vi "Obtain NI Settings UL.vi"(11 "Cluster INFO":T1={"Coefficenti P2"={"Af"=0.0, "Bf"=0.0, "Cf"=0.0, "Df"=0.0, "Ef"=0.0, "Ff"=0.0, "Gf"=0.0, "Hf"=0.0, "Jf"=0.0, "Kf"=0.0, "If"=0.0, "Ar"=0.0, "Br"=0.0, "Cr"=0.0, "Dr"=0.0, "Er"=0.0, "Fr"=0.0, "Gr"=0.0, "Hr"=0.0, "Jr"=0.0, "Kr"=0.0, "Ir"=0.0}, "Cluster settaggi wattmetro"={"Wattmetro"=enum."No Selection", "Alimentazione"=enum."Radio Selection 1"}, "SET RPM"=0.0, "SET TEMP"=0.0, "IMPOSTAZIONI INGRESSI UL"={"SALVA"=FALSE, "CARICA"=FALSE, "APPLICA"=FALSE, "Q1"={"Range"=0.0, "Offset"=0.0, "Medie"=0}, "Q2"={"Range"=0.0, "Offset"=0.0, "Medie"=0}, "Q3"={"Range"=0.0, "Offset"=0.0, "Medie"=0}, "P1"={"Range"=0.0, "Offset"=0.0, "Medie"=0}, "P2"={"Range"=0.0, "Offset"=0.0, "Medie"=0}, "P3"={"Range"=0.0, "Offset"=0.0, "Medie"=0}, "N"={"Range"=0.0, "Offset"=0.0, "Medie"=0}, "Tq"={"Range"=0.0, "Offset"=0.0, "Medie"=0}, "T"={"Range"=0.0, "Offset"=0.0, "Medie"=0}, "PORTATA PRINCIPALE"=0, "PORTATA SECONDARIA"=0, "PRESSIONE ASPIRAZIONE"=0, "PRESSIONE MANDATA"=0, "RPM"=0, "differenziale?"=FALSE}, "IMPOSTAZIONI INGRESSI NM"={"SALVA"=FALSE, "CARICA"=FALSE, "APPLICA"=FALSE, "Q1"={"Range"=0.0, "Offset"=0.0, "Medie"=0}, "Q2"={"Range"=0.0, "Offset"=0.0, "Medie"=0}, "Q3"={"Range"=0.0, "Offset"=0.0, "Medie"=0}, "Q4"={"Range"=0.0, "Offset"=0.0, "Medie"=0}, "Q5"={"Range"=0.0, "Offset"=0.0, "Medie"=0}, "Q6"={"Range"=0.0, "Offset"=0.0, "Medie"=0}, "Q7"={"Range"=0.0, "Offset"=0.0, "Medie"=0}, "Q8"={"Range"=0.0, "Offset"=0.0, "Medie"=0}, "Q9"={"Range"=0.0, "Offset"=0.0, "Medie"=0}, "Q10"={"Range"=0.0, "Offset"=0.0, "Medie"=0}, "P1"={"Range"=0.0, "Offset"=0.0, "Medie"=0}, "P2"={"Range"=0.0, "Offset"=0.0, "Medie"=0}, "P3"={"Range"=0.0, "Offset"=0.0, "Medie"=0}, "P4"={"Range"=0.0, "Offset"=0.0, "Medie"=0}, "P5"={"Range"=0.0, "Offset"=0.0, "Medie"=0}, "P6"={"Range"=0.0, "Offset"=0.0, "Medie"=0}, "P7"={"Range"=0.0, "Offset"=0.0, "Medie"=0}, "P8"={"Range"=0.0, "Offset"=0.0, "Medie"=0}, "P9"={"Range"=0.0, "Offset"=0.0, "Medie"=0}, "P10"={"Range"=0.0, "Offset"=0.0, "Medie"=0}, "N1(T)"={"Range"=0.0, "Offset"=0.0, "Medie"=0}, "N2(T)"={"Range"=0.0, "Offset"=0.0, "Medie"=0}, "N3(T)"={"Range"=0.0, "Offset"=0.0, "Medie"=0}, "Tq1"={"Range"=0.0, "Offset"=0.0, "Medie"=0}, "Tq2"={"Range"=0.0, "Offset"=0.0, "Medie"=0}, "Tq3"={"Range"=0.0, "Offset"=0.0, "Medie"=0}, "RM1"={"Range"=0.0, "Offset"=0.0, "Medie"=0}, "RM2"={"Range"=0.0, "Offset"=0.0, "Medie"=0}, "RM3"={"Range"=0.0, "Offset"=0.0, "Medie"=0}, "T1"={"Range"=0.0, "Offset"=0.0, "Medie"=0}, "T2"={"Range"=0.0, "Offset"=0.0, "Medie"=0}, "T3"={"Range"=0.0, "Offset"=0.0, "Medie"=0}, "T4"={"Range"=0.0, "Offset"=0.0, "Medie"=0}, "T5"={"Range"=0.0, "Offset"=0.0, "Medie"=0}, "T6"={"Range"=0.0, "Offset"=0.0, "Medie"=0}, "T7"={"Range"=0.0, "Offset"=0.0, "Medie"=0}, "T8"={"Range"=0.0, "Offset"=0.0, "Medie"=0}, "Liv."={"Range"=0.0, "Offset"=0.0, "Medie"=0}, "Pbar"={"Range"=0.0, "Offset"=0.0, "Medie"=0}, "PORTATA\nPRINCIPALE"=0, "PORTATA\nSECONDARIA"=0, "PRESSIONE\nASPIRAZIONE"=0, "PRESSIONE\nMANDATA"=0, "RPM"=0, "differenziale?"=FALSE}, "Costanti collaudo"={"P [bar]"=0.0, "T amb. [°C]"=0.0, "Umidità [%]"=0.0}, "Condizione P2"=enum."Radio Selection 1", "Array linee"=[{"portata"=0, "Hasp"=0, "Hmand"=1, "Torsiometro"=0, "rpm"=0, "Hdiff?"=FALSE, "T amb"=0, "Indici valvole"=[0, 1], "Nome"="Elettropompa", "Sommersa?"=FALSE}, {"portata"=1, "Hasp"=0, "Hmand"=0, "Torsiometro"=0, "rpm"=0, "Hdiff?"=FALSE, "T amb"=0, "Indici valvole"=[0, 1], "Nome"="Sommersa", "Sommersa?"=TRUE}], "Array valvole linee avvio/fermata"=[], "Linea selezionata"=0.0, "Tolleranze croci"={"Q"=0.0, "Htot"=0.0, "Ptot"=0.0, "EtaP"=0.0}, "Sett T e R"={"Tamb[°C]"=0.0, "Ru-w"=0.0, "Rmarcia"=0.0, "Raux"=0.0, "Tamb Freddo[°C]"=0.0, "Ru-w freddo"=0.0, "Rmarcia freddo"=0.0, "Raux freddop"=0.0, "TC1"=0.0, "TC2"=0.0, "TC3"=0.0, "TC4"=0.0, "TC5"=0.0, "TC6"=0.0, "TC7"=0.0, "TC8"=0.0}, "Nomi valvole prop sistema"=[], "Calcolo P2"=enum."Torsiometro", "Rendimento motore"=0.0, "curva rendimento"=[], "Coeff motore"={"a5"=0.0, "a4"=0.0, "a3"=0.0, "a2"=0.0, "a1"=0.0, "a0"=0.0, "P1max"=0.0, "P1min"=0.0}} {"IMPOSTAZIONI INGRESSI NM"."T8"."Medie" min=1 step=1; "IMPOSTAZIONI INGRESSI NM"."T7"."Medie" min=1 step=1; "IMPOSTAZIONI INGRESSI NM"."T6"."Medie" min=1 step=1; "IMPOSTAZIONI INGRESSI NM"."T5"."Medie" min=1 step=1; "IMPOSTAZIONI INGRESSI NM"."T4"."Medie" min=1 step=1; "IMPOSTAZIONI INGRESSI NM"."T3"."Medie" min=1 step=1; "IMPOSTAZIONI INGRESSI NM"."RM3"."Medie" min=1 step=1; "IMPOSTAZIONI INGRESSI NM"."Tq3"."Medie" min=1 step=1; "IMPOSTAZIONI INGRESSI NM"."Tq2"."Medie" min=1 step=1; "IMPOSTAZIONI INGRESSI NM"."N3(T)"."Medie" min=1 step=1; "IMPOSTAZIONI INGRESSI NM"."N2(T)"."Medie" min=1 step=1; "IMPOSTAZIONI INGRESSI NM"."P10"."Medie" min=1 step=1; "IMPOSTAZIONI INGRESSI NM"."P9"."Medie" min=1 step=1; "IMPOSTAZIONI INGRESSI NM"."P8"."Medie" min=1 step=1; "IMPOSTAZIONI INGRESSI NM"."P7"."Medie" min=1 step=1; "IMPOSTAZIONI INGRESSI NM"."P6"."Medie" min=1 step=1; "IMPOSTAZIONI INGRESSI NM"."P5"."Medie" min=1 step=1; "IMPOSTAZIONI INGRESSI NM"."Q10"."Medie" min=1 step=1; "IMPOSTAZIONI INGRESSI NM"."Q9"."Medie" min=1 step=1; "IMPOSTAZIONI INGRESSI NM"."Q8"."Medie" min=1 step=1; "IMPOSTAZIONI INGRESSI NM"."Q7"."Medie" min=1 step=1; "IMPOSTAZIONI INGRESSI NM"."Q6"."Medie" min=1 step=1; "IMPOSTAZIONI INGRESSI NM"."Q5"."Medie" min=1 step=1; "IMPOSTAZIONI INGRESSI NM"."Pbar"."Medie" min=1 step=1; "IMPOSTAZIONI INGRESSI NM"."Liv."."Medie" min=1 step=1; "IMPOSTAZIONI INGRESSI NM"."RM2"."Medie" min=1 step=1; "IMPOSTAZIONI INGRESSI NM"."RM1"."Medie" min=1 step=1; "IMPOSTAZIONI INGRESSI NM"."T2"."Medie" min=1 step=1; "IMPOSTAZIONI INGRESSI NM"."P4"."Medie" min=1 step=1; "IMPOSTAZIONI INGRESSI NM"."Q4"."Medie" min=1 step=1; "IMPOSTAZIONI INGRESSI NM"."RPM" items=["TESTO", "TORSIOMETRO", "OTTICA"]; "IMPOSTAZIONI INGRESSI NM"."PRESSIONE\nMANDATA" items=["P1", "P2", "P3", "P4"]; "IMPOSTAZIONI INGRESSI NM"."PRESSIONE\nASPIRAZIONE" items=["P1", "P2", "P3", "P4"]; "IMPOSTAZIONI INGRESSI NM"."PORTATA\nSECONDARIA" items=["Q1", "Q2", "Q3", "Q4"]; "IMPOSTAZIONI INGRESSI NM"."PORTATA\nPRINCIPALE" items=["LINEA ELETTROPOMPA", "LINEA SOMMERSA"]; "IMPOSTAZIONI INGRESSI NM"."T1"."Medie" min=1 step=1; "IMPOSTAZIONI INGRESSI NM"."Tq1"."Medie" min=1 step=1; "IMPOSTAZIONI INGRESSI NM"."N1(T)"."Medie" min=1 step=1; "IMPOSTAZIONI INGRESSI NM"."P3"."Medie" min=1 step=1; "IMPOSTAZIONI INGRESSI NM"."P2"."Medie" min=1 step=1; "IMPOSTAZIONI INGRESSI NM"."P1"."Medie" min=1 step=1; "IMPOSTAZIONI INGRESSI NM"."Q3"."Medie" min=1 step=1; "IMPOSTAZIONI INGRESSI NM"."Q2"."Medie" min=1 step=1; "IMPOSTAZIONI INGRESSI NM"."Q1"."Medie" min=1 step=1; "IMPOSTAZIONI INGRESSI UL"."RPM" items=["TESTO", "TORSIOMETRO", "OTTICA"]; "IMPOSTAZIONI INGRESSI UL"."PRESSIONE MANDATA" items=["P1", "P2", "P3"]; "IMPOSTAZIONI INGRESSI UL"."PRESSIONE ASPIRAZIONE" items=["P1", "P2", "P3"]; "IMPOSTAZIONI INGRESSI UL"."PORTATA SECONDARIA" items=["Q1", "Q2", "Q3"]; "IMPOSTAZIONI INGRESSI UL"."PORTATA PRINCIPALE" items=["Q1", "Q2", "Q3"]; "IMPOSTAZIONI INGRESSI UL"."T"."Medie" min=1 step=1; "IMPOSTAZIONI INGRESSI UL"."Tq"."Medie" min=1 step=1; "IMPOSTAZIONI INGRESSI UL"."N"."Medie" min=1 step=1; "IMPOSTAZIONI INGRESSI UL"."P3"."Medie" min=1 step=1; "IMPOSTAZIONI INGRESSI UL"."P2"."Medie" min=1 step=1; "IMPOSTAZIONI INGRESSI UL"."P1"."Medie" min=1 step=1; "IMPOSTAZIONI INGRESSI UL"."Q3"."Medie" min=1 step=1; "IMPOSTAZIONI INGRESSI UL"."Q2"."Medie" min=1 step=1; "IMPOSTAZIONI INGRESSI UL"."Q1"."Medie" min=1 step=1}) -> (1 "Campioni medie":u8[](array[numeric]), 3 "Array Settings":dbl[](array[numeric]))   [LabVIEW 2016]
uses:
  TypeDef/Cluster INFO.ctl
  TypeDef/WT SELECTION.ctl
  TypeDef/ALIM SELECTION.ctl
  TypeDef/cDAQ Settings UL.ctl
  TypeDef/SETUP INGRESSO.ctl
  TypeDef/cDAQ Settings NM.ctl
  TypeDef/Definizione linea.ctl
  TypeDef/sett T e R.ctl
panel:
  # "Freddo"
  # "Regime"
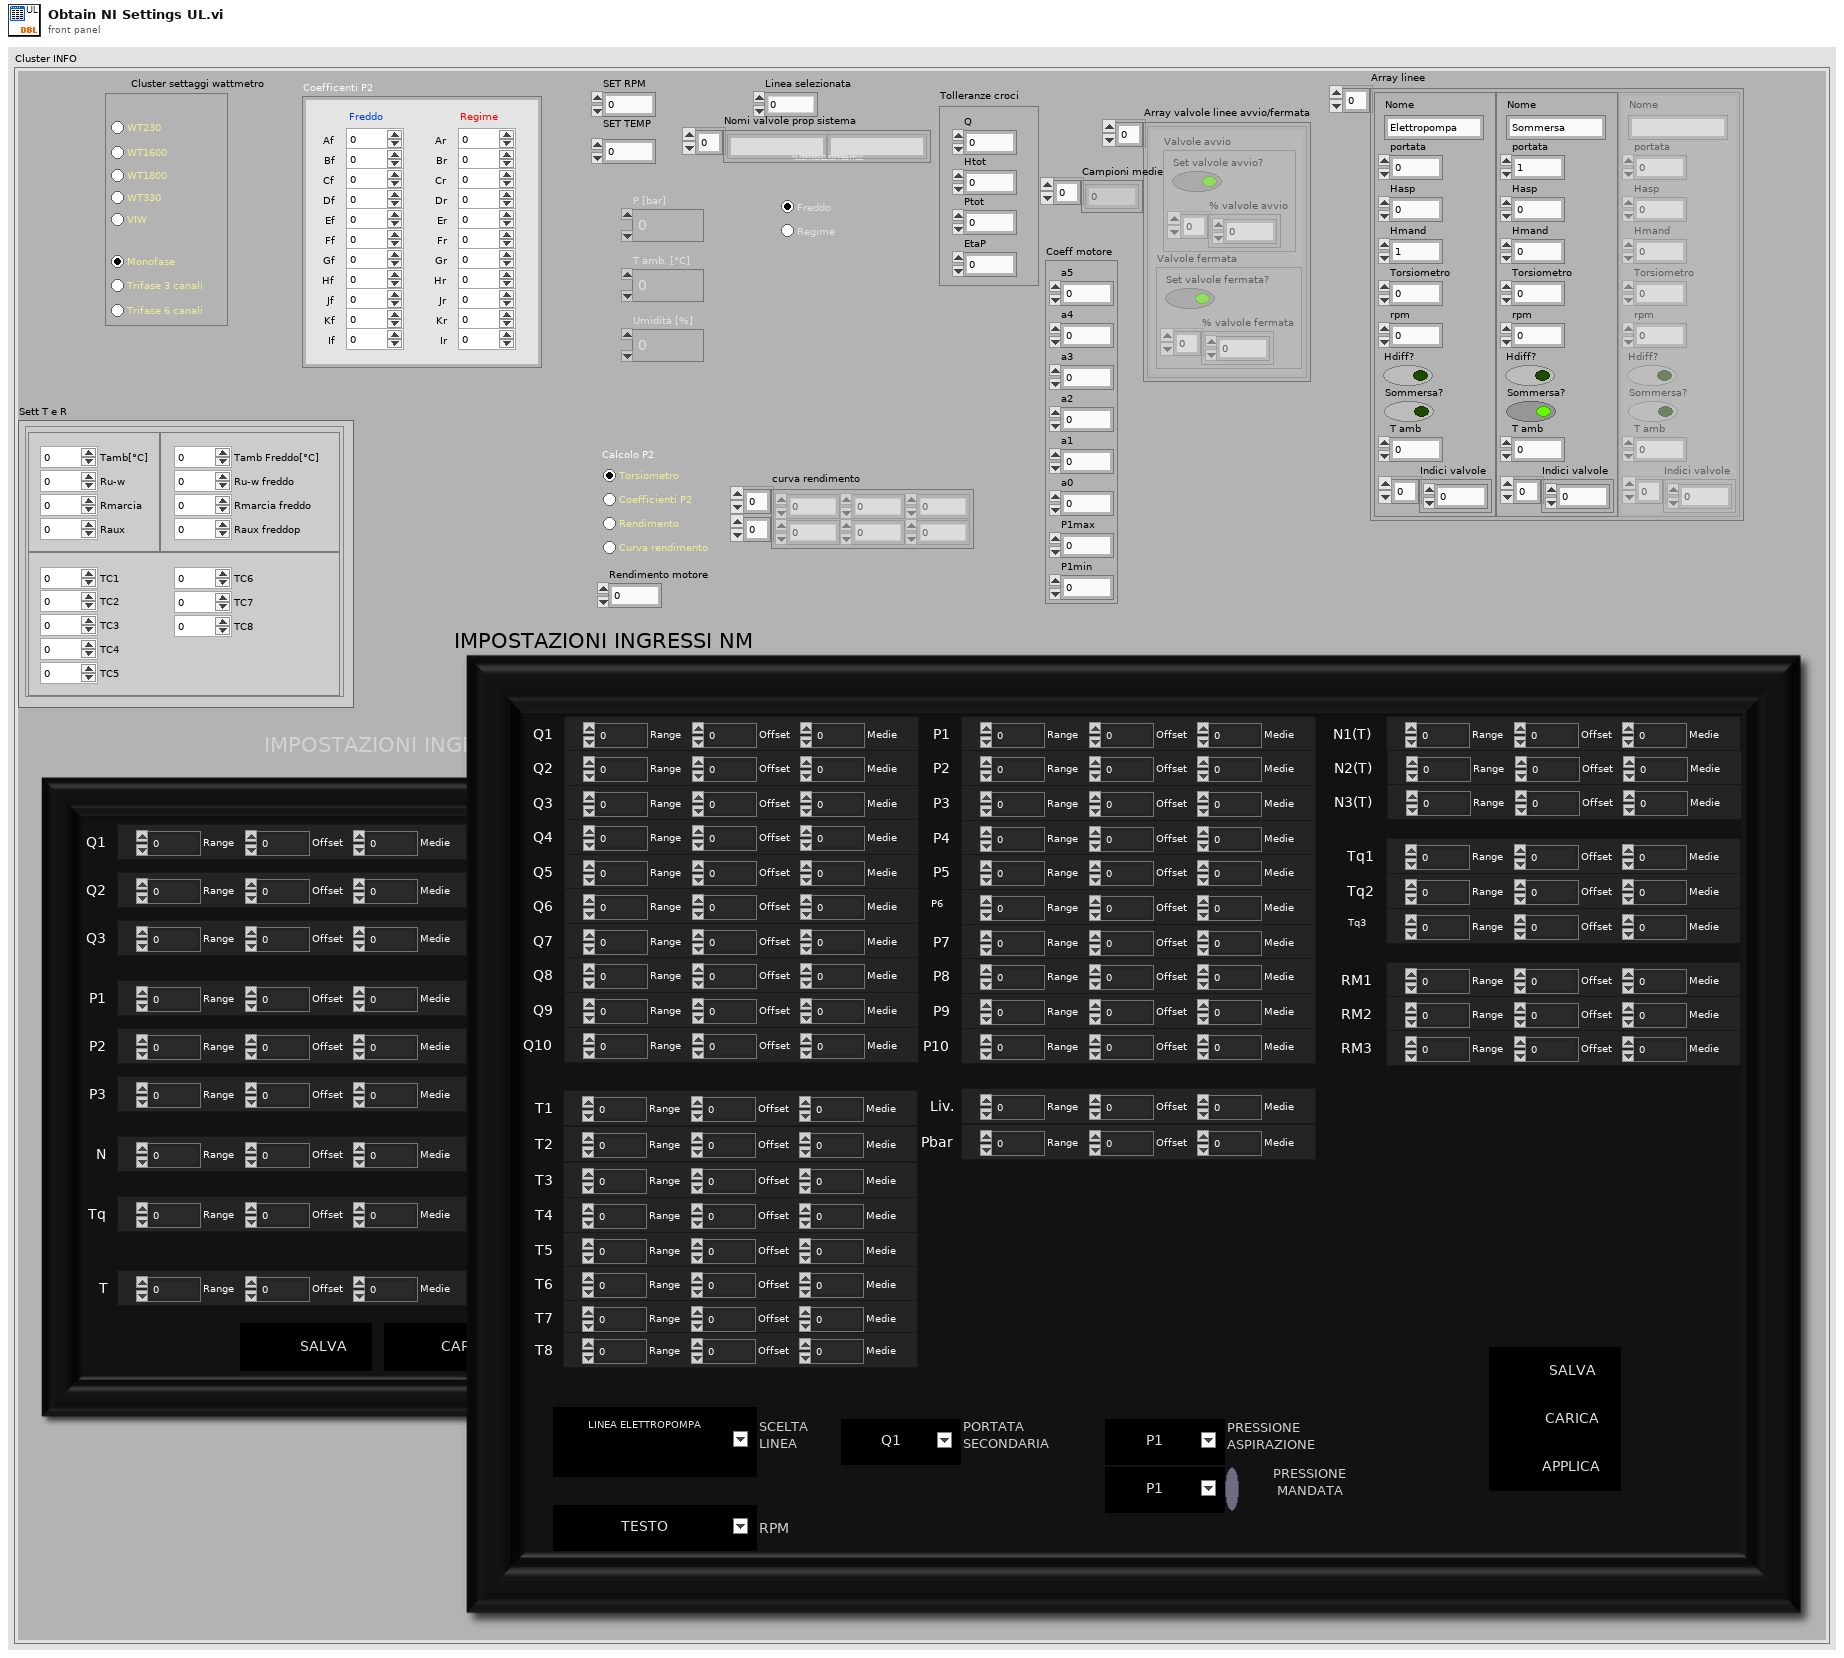
[diagram p1: front panel]
types:
  T1 = typedef "Cluster INFO.ctl" = cluster{"Coefficenti P2":cluster{"Af":dbl, "Bf":dbl, "Cf":dbl, "Df":dbl, "Ef":dbl, "Ff":dbl, "Gf":dbl, "Hf":dbl, "Jf":dbl, "Kf":dbl, "If":dbl, "Ar":dbl, "Br":dbl, "Cr":dbl, "Dr":dbl, "Er":dbl, "Fr":dbl, "Gr":dbl, "Hr":dbl, "Jr":dbl, "Kr":dbl, "Ir":dbl}, "Cluster settaggi wattmetro":cluster{"Wattmetro":T2, "Alimentazione":T3}, "SET RPM":dbl, "SET TEMP":dbl, "IMPOSTAZIONI INGRESSI UL":T4, "IMPOSTAZIONI INGRESSI NM":T6, "Costanti collaudo":cluster{"P [bar]":dbl, "T amb. [°C]":dbl, "Umidità [%]":dbl}, "Condizione P2":enum32{"Radio Selection 1", "Radio Selection 2"}, "Array linee":T7[], "Array valvole linee avvio/fermata":cluster{"Valvole avvio":cluster{"Set valvole avvio?":bool, "% valvole avvio":dbl[]}, "Valvole fermata":cluster{"Set valvole fermata?":bool, "% valvole fermata":dbl[]}}[], "Linea selezionata":dbl, "Tolleranze croci":cluster{"Q":dbl, "Htot":dbl, "Ptot":dbl, "EtaP":dbl}, "Sett T e R":T8, "Nomi valvole prop sistema":string[], "Calcolo P2":enum32{"Torsiometro", "coeff p2", "Rendimento", "Curva rend"}, "Rendimento motore":dbl, "curva rendimento":dbl[][], "Coeff motore":cluster{"a5":dbl, "a4":dbl, "a3":dbl, "a2":dbl, "a1":dbl, "a0":dbl, "P1max":dbl, "P1min":dbl}}
  T2 = typedef "WT SELECTION.ctl" = enum32{"No Selection", "WT230", "WT1600", "WT1800", "WT330", "VIW"}
  T3 = typedef "ALIM SELECTION.ctl" = enum32{"Radio Selection 1", "Radio Selection 2", "Radio Selection 3"}
  T4 = typedef "cDAQ Settings UL.ctl" = cluster{"SALVA":bool, "CARICA":bool, "APPLICA":bool, "Q1":T5, "Q2":T5, "Q3":T5, "P1":T5, "P2":T5, "P3":T5, "N":T5, "Tq":T5, "T":T5, "PORTATA PRINCIPALE":u16, "PORTATA SECONDARIA":u16, "PRESSIONE ASPIRAZIONE":u16, "PRESSIONE MANDATA":u16, "RPM":u16, "differenziale?":bool}
  T5 = typedef "SETUP INGRESSO.ctl" = cluster{"Range":dbl, "Offset":dbl, "Medie":u8}
  T6 = typedef "cDAQ Settings NM.ctl" = cluster{"SALVA":bool, "CARICA":bool, "APPLICA":bool, "Q1":T5, "Q2":T5, "Q3":T5, "Q4":T5, "Q5":T5, "Q6":T5, "Q7":T5, "Q8":T5, "Q9":T5, "Q10":T5, "P1":T5, "P2":T5, "P3":T5, "P4":T5, "P5":T5, "P6":T5, "P7":T5, "P8":T5, "P9":T5, "P10":T5, "N1(T)":T5, "N2(T)":T5, "N3(T)":T5, "Tq1":T5, "Tq2":T5, "Tq3":T5, "RM1":T5, "RM2":T5, "RM3":T5, "T1":T5, "T2":T5, "T3":T5, "T4":T5, "T5":T5, "T6":T5, "T7":T5, "T8":T5, "Liv.":T5, "Pbar":T5, "PORTATA\nPRINCIPALE":u16, "PORTATA\nSECONDARIA":u16, "PRESSIONE\nASPIRAZIONE":u16, "PRESSIONE\nMANDATA":u16, "RPM":u16, "differenziale?":bool}
  T7 = typedef "Definizione linea.ctl" = cluster{"portata":i32, "Hasp":i32, "Hmand":i32, "Torsiometro":i32, "rpm":i32, "Hdiff?":bool, "T amb":i32, "Indici valvole":i16[], "Nome":string, "Sommersa?":bool}
  T8 = typedef "sett T e R.ctl" = cluster{"Tamb[°C]":dbl, "Ru-w":dbl, "Rmarcia":dbl, "Raux":dbl, "Tamb Freddo[°C]":dbl, "Ru-w freddo":dbl, "Rmarcia freddo":dbl, "Raux freddop":dbl, "TC1":dbl, "TC2":dbl, "TC3":dbl, "TC4":dbl, "TC5":dbl, "TC6":dbl, "TC7":dbl, "TC8":dbl}
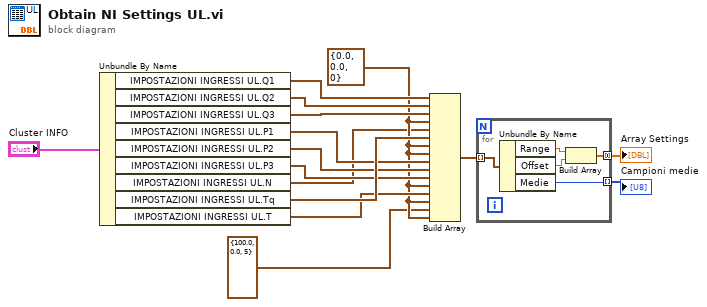
[diagram p0: block diagram]
diagram:
  w5 = T5 {"Range"=0.0, "Offset"=0.0, "Medie"=0} ("element")
  n1 = Unbundle By Name("Cluster INFO") -> ("IMPOSTAZIONI INGRESSI UL.Q1"=w13:T5, "IMPOSTAZIONI INGRESSI UL.Q2"=w12:T5, "IMPOSTAZIONI INGRESSI UL.Q3"=w11:T5, "IMPOSTAZIONI INGRESSI UL.P1"=w9:T5, "IMPOSTAZIONI INGRESSI UL.P2"=w8:T5, "IMPOSTAZIONI INGRESSI UL.P3"=w7:T5, "IMPOSTAZIONI INGRESSI UL.N"=w2:T5, "IMPOSTAZIONI INGRESSI UL.Tq"=w10:T5, "IMPOSTAZIONI INGRESSI UL.T"=w6:T5)
  n2 = Build Array(w13, w12, w11, w5, w2, w10, w5, w5, w9, w8, w7, w5, w6, w5, T5 {"Range"=100.0, "Offset"=0.0, "Medie"=5} ("element"), w5) -> (w4:T5[])
  n3 = for {
    tunnel: w4 -> [w20] mode=indexing
    tunnel: [w17] -> w15 mode=concatenating
    tunnel: [w16] -> w3 mode=indexing
    n4 = Unbundle By Name(w20) -> ("Range"=w19:dbl, "Offset"=w18:dbl, "Medie"=w16:u8)
    n5 = Build Array(w19, w18) -> (w17:dbl[])
  }
  "Array Settings" <- w15
  "Campioni medie" <- w3
